vi "Error Generator.vi"(8 "Error In":errorcluster, 10 "EZ430-Chronos Error Code":i32, 11 "EZ430-Chronos Ref":T1) -> (0 "Error Out":errorcluster, 3 "EZ430-Chronos Ref":T1)   [LabVIEW 2011, in "LVH-EZ430.lvlib"]
uses:
  <vilib>/LabVIEW Hacker/LabVIEW Interface for EZ430-Chronos/LVH-EZ430.lvlib
  <vilib>/LabVIEW Hacker/LabVIEW Interface for EZ430-Chronos/Private/Type Defs/EZ430-Chronos Ref.ctl
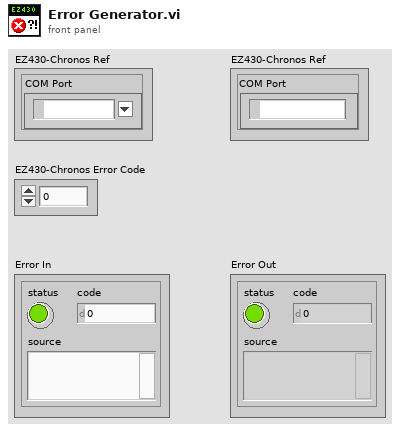
[diagram p1: front panel]
types:
  T1 = typedef "LVH-EZ430.lvlib/EZ430-Chronos Ref.ctl" = cluster{"COM Port":refnum<visa-resource-name>}
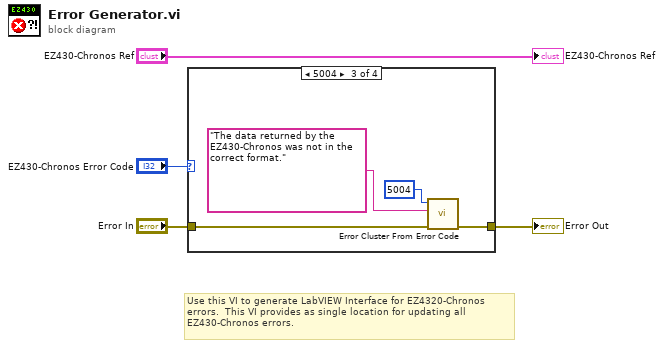
[diagram p0: block diagram]
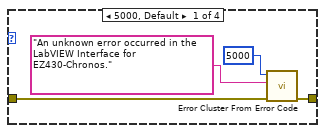
[diagram p2: hidden frame]
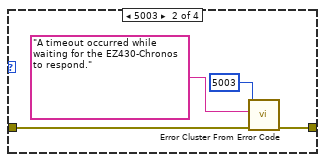
[diagram p3: hidden frame]
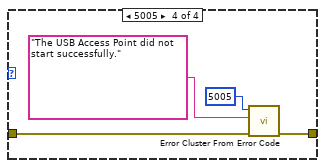
[diagram p4: hidden frame]
diagram:
  # "Use this VI to generate LabVIEW Interface for EZ4320-Chronos \nerrors.  This VI provides as single location for updating all \nEZ430-Chronos errors."
  n1 = case shown="5004" "EZ430-Chronos Error Code" {
    tunnel: "Error In" -> [w6 w10 w14 w18]
    tunnel: [w5 w11 w15 w19] -> w2
    frame 5000, Default {
      n2 = call <vilib>:"Error Cluster From Error Code.vi"("error in (no error)"=w6, "error message (\"\")"="An unknown error occurred in the LabVIEW Interface for EZ430-Chronos.", "error code (0)"=5000) -> ("error out"=w5:errorcluster)  [unwired: 6 in]
    }
    frame 5003 {
      n3 = call <vilib>:"Error Cluster From Error Code.vi"("error in (no error)"=w10, "error message (\"\")"="A timeout occurred while waiting for the EZ430-Chronos to respond." ("error message (\"\")"), "error code (0)"=5003) -> ("error out"=w11:errorcluster)  [unwired: 6 in]
    }
    frame 5004 {
      n4 = call <vilib>:"Error Cluster From Error Code.vi"("error in (no error)"=w14, "error message (\"\")"="The data returned by the EZ430-Chronos was not in the correct format." ("error message (\"\")"), "error code (0)"=5004) -> ("error out"=w15:errorcluster)  [unwired: 6 in]
    }
    frame 5005 {
      n5 = call <vilib>:"Error Cluster From Error Code.vi"("error in (no error)"=w18, "error message (\"\")"="The USB Access Point did not start successfully." ("error message (\"\")"), "error code (0)"=5005) -> ("error out"=w19:errorcluster)  [unwired: 6 in]
    }
  }
  "Error Out" <- w2
  "EZ430-Chronos Ref" <- "EZ430-Chronos Ref"
